vi "Create Transfer.vi"(4 "size":u64, 5 "id":i32, 6 "group offset":u64, 7 "channel blocks":T1[](array[typedef]) {"buffer offset" format="%d bytes"}, 8 "error in (no error)":errorcluster, 9 "String Buffer":refnum<class "Memory Buffer.lvclass">, 10 "Intermediate Buffer":refnum<class "Double Pointer.lvclass">, 11 "Inline Buffer":refnum<class "Double Pointer.lvclass">) -> (0 "error out":errorcluster, 3 "Transfer out":refnum<class "Transfer.lvclass">)   [LabVIEW 2017, in "Data Sharing Framework Core.lvlib" / "Data Sharing Framework Engine.lvlib" / "Transfer.lvclass"]
uses:
  Transfer.lvclass
  Internal/Memory/Memory Buffer/Memory Buffer.lvclass
  Internal/Memory/Double Pointer/Double Pointer.lvclass
  Internal/Type Definitions/DSF Runtime Channel Block.ctl
  Configuration/1.0.0/Public/Controls/DSF Data Type.ctl
  Transfer.lvclass/Transfer.ctl
  Data Sharing Framework Engine.lvlib
  Configuration/1.0.0/Data Sharing Framework Configuration.lvlib
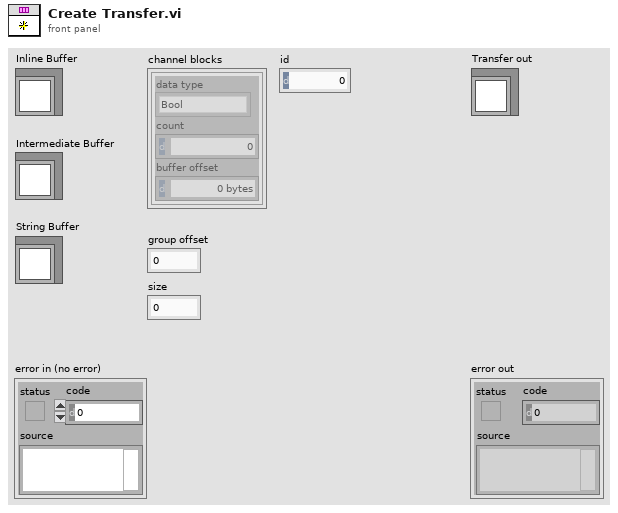
[diagram p1: front panel]
types:
  T1 = typedef "Data Sharing Framework Core.lvlib/Data Sharing Framework Engine.lvlib/DSF Runtime Channel Block.ctl" = cluster{"data type":T2, "count":u64, "buffer offset":u64}
  T2 = typedef "Data Sharing Framework Core.lvlib/Data Sharing Framework Configuration.lvlib/DSF Data Type.ctl" = enum8{"Bool", "SGL", "DBL", "I8", "I16", "I32", "I64", "U8", "U16", "U32", "U64"}
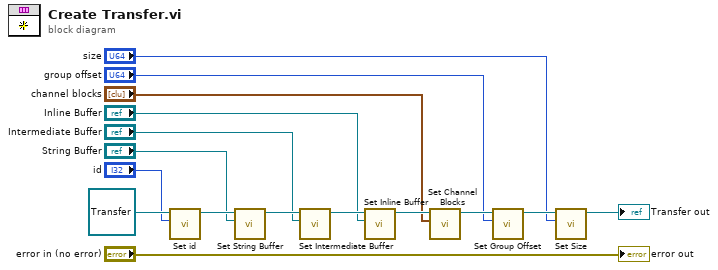
[diagram p0: block diagram]
diagram:
  n1 = call "Set id.vi"("id"="id", "Transfer in"=refnum<class "Transfer.lvclass"> refnum) -> ("Transfer out"=w16:refnum<class "Transfer.lvclass">)  [unwired: 9 in]
  n2 = call "Set String Buffer.vi"("Buffer"="String Buffer", "Transfer in"=w16) -> ("Transfer out"=w15:refnum<class "Transfer.lvclass">)  [unwired: 9 in]
  n3 = call "Set Intermediate Buffer.vi"("DBL Buffer"="Intermediate Buffer", "Transfer in"=w15) -> ("Transfer out"=w14:refnum<class "Transfer.lvclass">)  [unwired: 9 in]
  n4 = call "Set Inline Buffer.vi"("Inline Buffer"="Inline Buffer", "Transfer in"=w14) -> ("Transfer out"=w7:refnum<class "Transfer.lvclass">)  [unwired: 9 in]
  n5 = call "Set Channel Blocks.vi"("channel blocks"="channel blocks", "Transfer in"=w7) -> ("Transfer out"=w5:refnum<class "Transfer.lvclass">)  [unwired: 9 in]
  n6 = call "Set Group Offset.vi"("group offset"="group offset", "Transfer in"=w5) -> ("Transfer out"=w4:refnum<class "Transfer.lvclass">)  [unwired: 9 in]
  n7 = call "Set Size.vi"("engine size"="size", "Transfer in"=w4) -> ("Transfer out"=→"Transfer out":refnum<class "Transfer.lvclass">)  [unwired: 9 in]
  "error out" <- "error in (no error)"
